vi "Destroy Connection.vi"(8 "error in (no error)":errorcluster, 11 "connection reference":T1) -> (0 "error out":errorcluster)   [LabVIEW 2020, in "PostgreSQL Driver.lvlib"]
uses:
  PostgreSQL Driver.lvlib
  <vilib>/addons/database/Connection.llb/Conn ObjectReference.ctl
  <vilib>/addons/database/NI_Database_API.lvlib
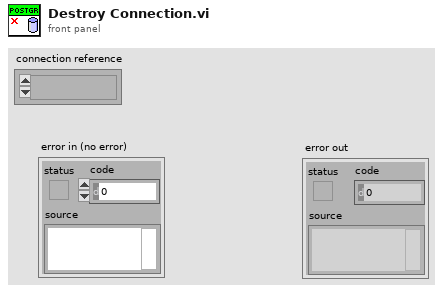
[diagram p1: front panel]
types:
  T1 = typedef "NI_Database_API.lvlib/Conn ObjectReference.ctl" = refnum<k1>
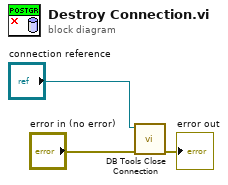
[diagram p0: block diagram]
diagram:
  n1 = call <vilib>:"DB Tools Close Connection.vi"("error in (no error)"="error in (no error)", "connection reference"="connection reference") -> ("error out"=→"error out":errorcluster)  [unwired: 5 in]
